vi "Write Class File Name.vi"(8 "error in (no error)":errorcluster, 10 "Class File Name":string, 11 "Generate From File in":refnum<class "Generate From File.lvclass">) -> (0 "error out":errorcluster, 3 "Generate From File out":refnum<class "Generate From File.lvclass">)   [LabVIEW 2011, in "Generate From File.lvclass"]
uses:
  Generate From File.lvclass
  Generate From File.lvclass/Generate From File.ctl
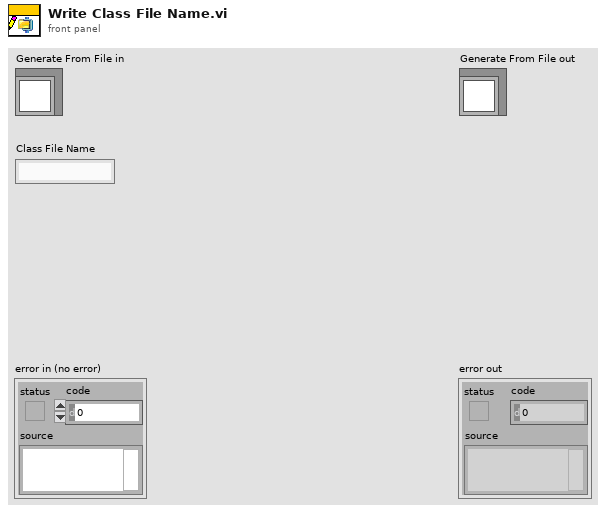
[diagram p1: front panel]
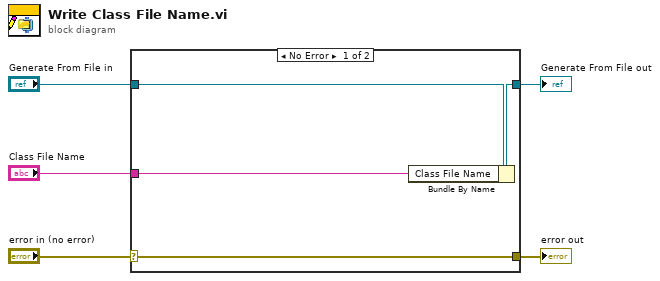
[diagram p0: block diagram]
diagram:
  n1 = case shown="No Error" "error in (no error)" {
    selector: "error in (no error)" -> [w9 w10]
    tunnel: [w9 w10] -> w4
    tunnel: [w7 w11] -> w2
    tunnel: "Generate From File in" -> [w8 w11]
    tunnel: "Class File Name" -> [w6 _]
    frame No Error {
      n2 = Bundle By Name(cluster=w8, "Class File Name"=w6) -> (w7:refnum<class "Generate From File.lvclass">)
    }
    frame Error {
    }
  }
  "error out" <- w4
  "Generate From File out" <- w2
